vi "Copy Inline to Async.vi"(8 "error in (no error)":errorcluster, 11 "Transfer Group in":refnum<class "Transfer Group.lvclass">) -> (0 "error out":errorcluster, 3 "Transfer Group out":refnum<class "Transfer Group.lvclass">)   [LabVIEW 2017, in "DSF Core.lvlib" / "Transfer Group.lvclass"]
uses:
  Transfer Group.lvclass
  Transfer Group.lvclass/Transfer Group.ctl
  Buffer/Buffers.lvclass
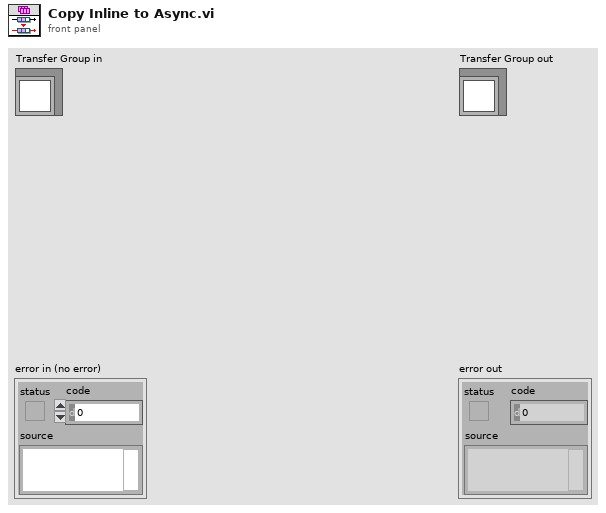
[diagram p1: front panel]
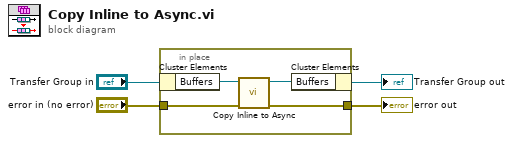
[diagram p0: block diagram]
diagram:
  n1 = in-place {
    in-place-border: "error in (no error)" -> [w6]
    in-place-border: [w5] -> w1
    n2 = in-place-cluster #1("Transfer Group in") -> ("Buffers"=w8:refnum<class "Buffers.lvclass">)
    n3 = call "Copy Inline to Async.vi"("error in (no error)"=w6, "Buffers in"=w8) -> ("error out"=w5:errorcluster, "Buffers out"=w7:refnum<class "Buffers.lvclass">)  [unwired: 8 in]
    n4 = in-place-cluster #1("Buffers"=w7) -> (→"Transfer Group out":refnum<class "Transfer Group.lvclass">)
  }
  "error out" <- w1
